vi "getSheetsName.vi"(8 "error in (no error)":errorcluster, 10 "filePath":string, 11 "reference in":refnum<class "python.lvclass">) -> (0 "error out":errorcluster, 2 "sheetsName":string[](array[string]), 3 "reference out":refnum<class "python.lvclass">)   [LabVIEW 2014, in "python.lvclass"]
uses:
  python.lvclass
  <vilib>/Utility/error.llb/DialogType.ctl
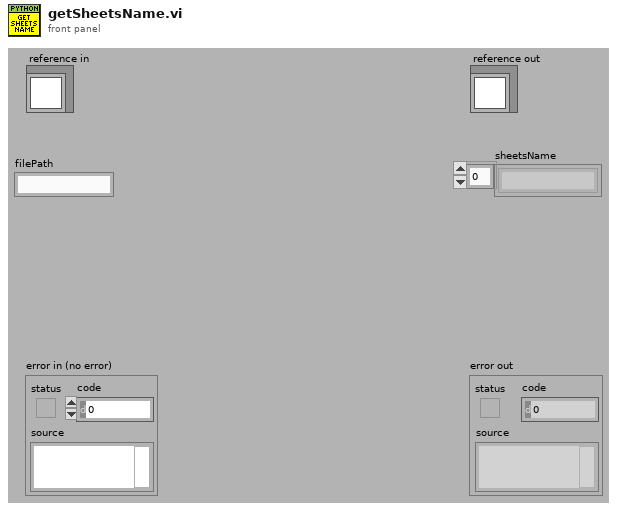
[diagram p1: front panel]
types:
  T1 = typedef "python.lvclass/ObjectAttributesRef.ctl" = refnum<data-value>
  T2 = typedef "python.lvclass/ObjectAttributes.ctl" = cluster{"MyAttribute":dbl, "workingDirectory":path}
  T3 = typedef "DialogType.ctl" = u16
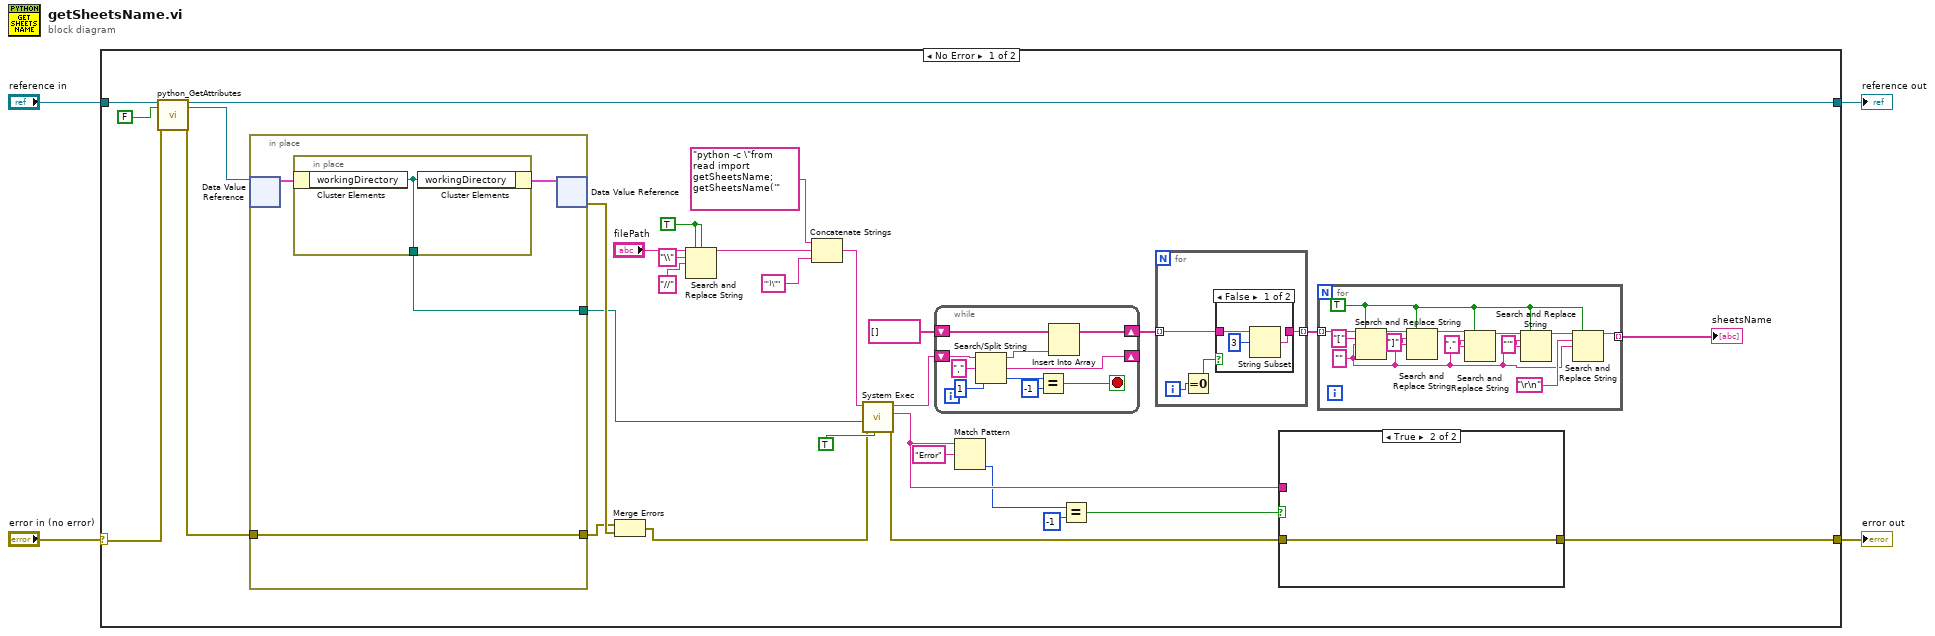
[diagram p0: block diagram]
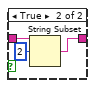
[diagram p2: hidden frame]
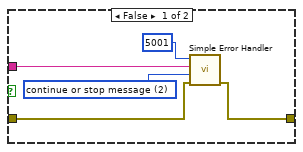
[diagram p3: hidden frame]
diagram:
  n1 = case shown="No Error" "error in (no error)" {
    selector: "error in (no error)" -> [w31 w81]
    tunnel: [w17 w81] -> w3
    tunnel: [w29 w80] -> w1
    tunnel: "reference in" -> [w33 w80]
    frame No Error {
      w12 = TRUE ("replace all? (F)")
      n2 = call "python_GetAttributes.vi"("reference in"=w33, "return data? (T)"=FALSE, "error in (no error)"=w31) -> ("reference out"=w29:refnum<class "python.lvclass">, "attributes ref"=w28:T1, "error out"=w30:errorcluster)  [unwired: 13 in, 1 out]
      n3 = in-place {
        in-place-border: w30 -> [w76]
        in-place-border: [w76] -> w34
        in-place-border: [w75] -> w26
        n4 = in-place-dvr #1(w28) -> (w77:T2)  [unwired: 1 out]
        n5 = in-place {
          in-place-border: [w79] -> w75
          n6 = in-place-cluster #2(w77) -> ("workingDirectory"=w79:path)
          n7 = in-place-cluster #2("workingDirectory"=w79) -> (w78:T2)
        }
        n8 = in-place-dvr #1(w78) -> (w35:errorcluster)  [unwired: 1 out]
      }
      n9 = Merge Errors(w34, w35) -> (w25:errorcluster)
      n10 = Search and Replace String(replace all?=w12, case sensitive?=w12, input string="filePath", search string="\\", replace string="//" ("search string")) -> (result string=w13:string)  [unwired: 3 in, 3 out]
      n11 = Concatenate Strings("python -c \"from read import getSheetsName; getSheetsName('" ("string"), w13, "')\"" ("string")) -> (w22:string)
      n12 = call <vilib>:"System Exec.vi"("run minimized? (F)"=TRUE, "error in (no error)"=w25, "working directory"=w26, "command line"=w22) -> ("error out"=w18:errorcluster, "standard error"=w11:string, "standard output"=w20:string)  [unwired: 2 in, 3 out]
      n13 = while {
        shift-right: [w73] -> w6
        shift-left: string[] [] -> [w74]
        shift-right: [w69] -> _
        shift-left: w20 -> [w72]
        stop <- w67 stop-if-true
        n14 = Search/Split String(string=w72, search string/char (-)=",", offset (0)=1) -> (substring before match=w71:string, match + rest of string=w69:string, offset of match=w68:i32)
        n15 = Equal?(x=w68, y=-1) -> (x = y?=w67:bool)
        n16 = Insert Into Array(array=w74, new element=w71) -> (w73:string[])  [unwired: 1 in]
      }
      n17 = Match Pattern(string=w11, regular expression="Error") -> (offset past match=w7:i32)  [unwired: 1 in, 3 out]
      n18 = Equal?(x=w7, y=-1 ("offset past match")) -> (x = y?=w8:bool)
      n19 = for {
        tunnel: w6 -> [w39] mode=indexing
        tunnel: [w38] -> w5 mode=indexing
        i -> [w37]
        n20 = Equal To 0?(x=w37) -> (x = 0?=w36:bool)
        n21 = case shown="False" w36 {
          tunnel: w39 -> [w42 w45]
          tunnel: [w40 w44] -> w38
          frame False {
            n22 = String Subset(string=w42, offset (0)=3) -> (substring=w40:string)  [unwired: 1 in]
          }
          frame True {
            n23 = String Subset(string=w45, offset (0)=2) -> (substring=w44:string)  [unwired: 1 in]
          }
        }
      }
      n24 = case shown="True" w8 {
        tunnel: w18 -> [w50 w51]
        tunnel: [w49 w51] -> w17
        tunnel: w11 -> [w47 _]
        frame False {
          w46 = T3 2 items=["no dialog", "OK message", "continue or stop message", "OK message + warnings", "continue/stop + warnings"] ("type of dialog (OK msg:1)")
          n25 = call <vilib>:"Simple Error Handler.vi"("error code (no error:0)"=5001, "error source (\" \")"=w47, "type of dialog (OK msg:1)"=w46, "error in (no error)"=w50) -> ("error out"=w49:errorcluster)  [unwired: 5 out]
        }
        frame True {
        }
      }
      n26 = for {
        tunnel: w5 -> [w64] mode=indexing
        tunnel: [w52] -> w19 mode=indexing
        w54 = TRUE ("replace all? (F)")
        w53 = "" ("replace string (\"\")")
        n27 = Search and Replace String(replace all?=w54, input string=w64, search string="[", replace string=w53) -> (result string=w62:string)  [unwired: 4 in, 3 out]
        n28 = Search and Replace String(replace all?=w54, input string=w62, search string="]", replace string=w53) -> (result string=w59:string)  [unwired: 4 in, 3 out]
        n29 = Search and Replace String(replace all?=w54, input string=w59, search string=",", replace string=w53) -> (result string=w57:string)  [unwired: 4 in, 3 out]
        n30 = Search and Replace String(replace all?=w54, input string=w57, search string="'", replace string=w53) -> (result string=w56:string)  [unwired: 4 in, 3 out]
        n31 = Search and Replace String(replace all?=w54, input string=w56, search string="\r\n", replace string=w53) -> (result string=w52:string)  [unwired: 4 in, 3 out]
      }
      "sheetsName" <- w19
    }
    frame Error {
    }
  }
  "error out" <- w3
  "reference out" <- w1
